vi "Frame_acquisition_server.vi"() -> ()   [LabVIEW 2026]
panel:
  in  "Acq Trigger":bool
  out "T":dbl[][](array[numeric])
  out "Intensity Graph":dbl[][](graph)
  out "DeltaT":dbl[][](array[numeric])
  in  "N":dbl
  # "IMAGE SETTINGS"
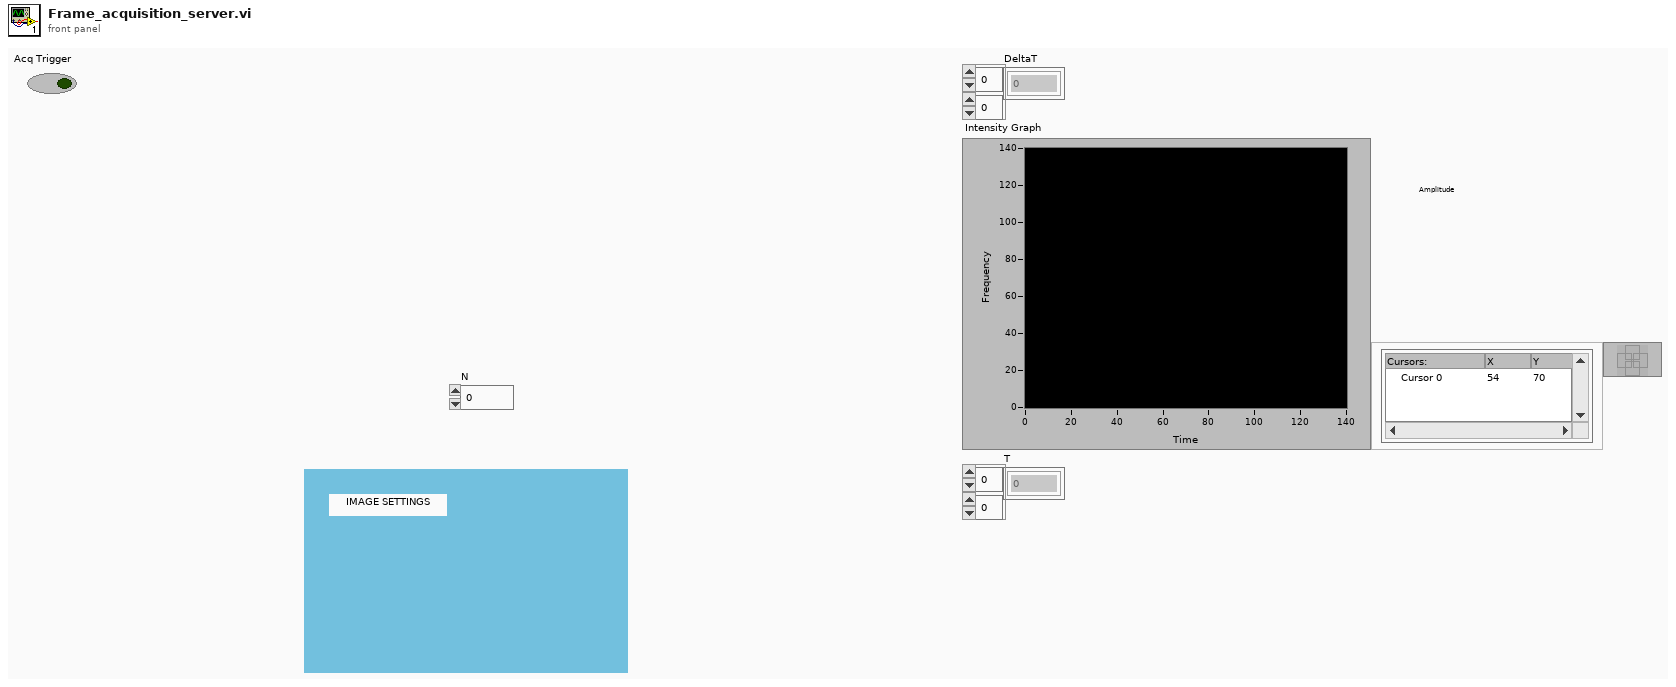
[diagram p1: front panel]
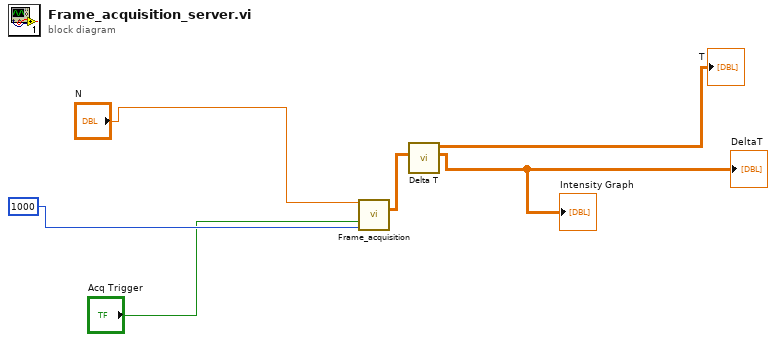
[diagram p0: block diagram]
diagram:
  n1 = call "Frame_acquisition.vi"("Frames"="N", "Acq Trigger?"="Acq Trigger", "Timeout"=1000) -> ("FrameData"=w6:dbl[][][])  [unwired: 11 in, 1 out]
  n2 = call "Delta T.vi"("FrameData"=w6) -> ("Delta T"=→"DeltaT" →"Intensity Graph":dbl[][], "T"=→"T":dbl[][])  [unwired: 7 in, 2 out]
